vi "Lab Panel V5.22.vi"() -> ()   [LabVIEW 2013] (continued)
                    n1469 = Greater Or Equal?(x=w2760, y=w2759) -> (x >= y?=w2761:bool)
                    n1470 = case shown="True" w2761 {
                      tunnel: w2757 -> [w2764 _]
                      tunnel: w2756 -> [w2763 _]
                      tunnel: w2755 -> [w2762 _]
                      frame True {
                        n1471 = stacked-sequence {
                          tunnel: w2764 -> [w2767 _]
                          tunnel: w2763 -> [_ w2772]
                          tunnel: w2762 -> [w2765 _]
                          frame #0 {
                            n1472 = Build Array("T-RISE") -> (w2769:string[])
                            n1473 = Build Array(w2767) -> (w2768:dbl[])
                            n1474 = TDMS Write(0:w2765, 5:"TEST PASS", 7:w2769, 9:w2768) -> (15:w2771:errorcluster)  [unwired: 2 in, 3 out]
                            n1475 = local write "data file error"(w2771) -> ()
                          }
                          frame #1 {
                            n1476 = Bundle(cluster=w2772, "STATUS"="T-RISE PASS") -> (w2774:T4)  [unwired: 2 in]
                            n1477 = local write "RESULT LAB05-1"(TRUE) -> ()
                            n1478 = local write "DISP LAB05-1"(w2774) -> ()
                          }
                        }
                      }
                      frame False {
                      }
                    }
                  }
                }
              }
              frame #9 {
                # "LAB05-2"
                n1479 = Equal?(x=w2777, y=2) -> (x = y?=w2780:bool)
                n1480 = local read "DISP LAB05-2"() -> (w2782:T4)
                n1481 = Unbundle(w2782) -> ("STATUS"=w2783:string)  [unwired: 2 out]
                n1482 = Equal?(x=w2783, y="RUN") -> (x = y?=w2779:bool)
                n1483 = And(x=w2779, y=w2780) -> (x .and. y?=w2778:bool)
                n1484 = case shown="True" w2778 {
                  tunnel: w2782 -> [_ w2786]
                  tunnel: w2776 -> [_ w2789]
                  frame False {
                  }
                  frame True {
                    n1485 = local read "SET LAB05-2"() -> (w2788:T5)
                    n1486 = local read "TDMS LAB05-2"() -> (w2785:refnum<k34>)
                    n1487 = Unbundle(w2786) -> ("CYCLE"=w2790:dbl)  [unwired: 2 out]
                    n1488 = Unbundle(w2788) -> ("T-RISE mins"=w2787:dbl)  [unwired: 4 out]
                    n1489 = Greater Or Equal?(x=w2790, y=w2789) -> (x >= y?=w2791:bool)
                    n1490 = case shown="True" w2791 {
                      tunnel: w2787 -> [w2794 _]
                      tunnel: w2786 -> [w2793 _]
                      tunnel: w2785 -> [w2792 _]
                      frame True {
                        n1491 = stacked-sequence {
                          tunnel: w2794 -> [w2797 _]
                          tunnel: w2793 -> [_ w2802]
                          tunnel: w2792 -> [w2795 _]
                          frame #0 {
                            n1492 = Build Array("T-RISE") -> (w2799:string[])
                            n1493 = Build Array(w2797) -> (w2798:dbl[])
                            n1494 = TDMS Write(0:w2795, 5:"TEST PASS", 7:w2799, 9:w2798) -> (15:w2801:errorcluster)  [unwired: 2 in, 3 out]
                            n1495 = local write "data file error"(w2801) -> ()
                          }
                          frame #1 {
                            n1496 = Bundle(cluster=w2802, "STATUS"="T-RISE PASS") -> (w2804:T4)  [unwired: 2 in]
                            n1497 = local write "RESULT LAB05-2"(TRUE) -> ()
                            n1498 = local write "DISP LAB05-2"(w2804) -> ()
                          }
                        }
                      }
                      frame False {
                      }
                    }
                  }
                }
              }
            }
          }
          frame #6 {
            # "end test & close test files"
            n1499 = local read "MAIL SETTINGS"() -> (w2810:T7)
            n1500 = Unbundle(w2810) -> ("OUT SERVER ADDRESS"=w2809:string, "FROM ACCOUNT"=w2808:string)  [unwired: 5 out]
            n1501 = stacked-sequence {
              tunnel: w2820 -> [_ _ _ _ _ _ _ _ _ _]
              tunnel: w2821 -> [_ _ _ _ _ _ _ _ _ _]
              tunnel: w2819 -> [_ _ _ _ _ _ _ _ _ _]
              tunnel: w2818 -> [_ _ _ _ _ _ _ _ _ _]
              tunnel: w2817 -> [_ _ _ _ _ _ _ _ _ _]
              tunnel: w2816 -> [_ _ _ _ _ _ _ _ _ _]
              tunnel: w2815 -> [_ _ _ _ _ _ _ _ _ _]
              tunnel: w2814 -> [_ _ _ _ _ _ _ _ _ _]
              tunnel: w2813 -> [_ _ _ _ _ _ _ _ _ _]
              tunnel: w2812 -> [_ _ _ _ _ _ _ _ _ _]
              tunnel: w2809 -> [w2825 w2877 w2925 w2972 w3019 w3066 w3113 w3160 w3207 w3254]
              tunnel: w2808 -> [w2824 w2876 w2924 w2971 w3018 w3065 w3112 w3159 w3206 w3253]
              tunnel: "Mail Test File To:" -> [w2823 w2875 w2923 w2970 w3017 w3064 w3111 w3158 w3205 w3252]
              tunnel: "Mail Test Fail" -> [w2822 w2874 w2922 w2969 w3016 w3063 w3110 w3157 w3204 w3251]
              frame #0 {
                # "LAB01-1"
                n1502 = local read "DISP LAB01-1"() -> (w2829:T4)
                n1503 = local read "run lab01-1"() -> (w2826:bool)
                n1504 = local read "TDMS LAB01-1"() -> (w2827:refnum<k34>)
                n1505 = Unbundle(w2829) -> ("CYCLE"=w2830:dbl, "STATUS"=w2828:string)  [unwired: 1 out]
                n1506 = case shown="True" w2826 {
                  tunnel: w2830 -> [_ w2836]
                  tunnel: w2829 -> [_ w2838]
                  tunnel: w2828 -> [_ w2835]
                  tunnel: w2827 -> [_ w2837]
                  tunnel: w2825 -> [_ w2834]
                  tunnel: w2824 -> [_ w2833]
                  tunnel: w2823 -> [_ w2832]
                  tunnel: w2822 -> [_ w2831]
                  frame False {
                  }
                  frame True {
                    n1507 = Not Equal?(x=w2835, y="RUN") -> (x != y?=w2839:bool)
                    n1508 = Greater?(x=w2836, y=2.0) -> (0:w2841:bool)
                    n1509 = And(x=w2841, y=w2839) -> (x .and. y?=w2840:bool)
                    n1510 = case shown="True" w2840 {
                      tunnel: w2838 -> [_ w2851]
                      tunnel: w2837 -> [_ w2850]
                      tunnel: w2836 -> [_ w2849]
                      tunnel: w2835 -> [_ w2848]
                      tunnel: w2834 -> [_ w2847]
                      tunnel: w2833 -> [_ w2846]
                      tunnel: w2832 -> [_ w2845]
                      tunnel: w2831 -> [_ w2844]
                      frame False {
                      }
                      frame True {
                        n1511 = stacked-sequence {
                          tunnel: w2851 -> [w2855 _ _]
                          tunnel: w2850 -> [_ w2857 _]
                          tunnel: w2849 -> [_ _ _]
                          tunnel: w2848 -> [_ _ w2863]
                          tunnel: w2847 -> [_ _ w2862]
                          tunnel: w2846 -> [_ _ w2861]
                          tunnel: w2845 -> [_ _ w2860]
                          tunnel: w2844 -> [_ _ w2859]
                          frame #0 {
                            w2852 = FALSE
                            n1512 = local write "mail control"("END") -> ()
                            n1513 = Bundle(cluster=w2855) -> (w2854:T4)  [unwired: 3 in]
                            n1514 = local write "DISP LAB01-1"(w2854) -> ()
                            n1515 = local write "O/I  LAB01-1"(w2852) -> ()
                            n1516 = local write "run lab01-1"(w2852) -> ()
                            n1517 = local write "RUN LAB01-1"(w2852) -> ()
                          }
                          frame #1 {
                            n1518 = TDMS Close(11:w2857) -> (0:w2856:errorcluster)  [unwired: 1 in, 1 out]
                            n1519 = local write "data file error"(w2856) -> ()
                          }
                          frame #2 {
                            n1520 = stacked-sequence {
                              tunnel: "LAB01-1" -> [w2865 w2867 _]
                              tunnel: w2863 -> [_ w2873 _]
                              tunnel: w2862 -> [_ w2872 _]
                              tunnel: w2861 -> [_ w2871 _]
                              tunnel: w2860 -> [_ w2870 _]
                              tunnel: w2859 -> [_ w2869 _]
                              frame #0 {
                                n1521 = call "sub vi - defrag tdms v1.vi"("panel id"=w2865) -> ("error out"=w2864:errorcluster)  [unwired: 10 in]
                                n1522 = local write "data file error"(w2864) -> ()
                              }
                              frame #1 {
                                n1523 = Bundle("STATUS"=w2873, "OUT SERVER ADDRESS"=w2872, "FROM ACCOUNT"=w2871, "Mail Test File To:"=w2870, "Mail Test Fail"=w2869) -> (w2866:T25)  [unwired: 1 in]
                                n1524 = call "Save data file (pass-fail) v5.vi"("Input Cluster"=w2866, "panel id"=w2867) -> ("network file save error"=w2868:errorcluster)  [unwired: 8 in, 1 out]
                                n1525 = local write "data file error"(w2868) -> ()
                              }
                              frame #2 {
                              }
                            }
                          }
                        }
                      }
                    }
                  }
                }
              }
              frame #1 {
                # "LAB01-2"
                n1526 = local read "run lab01-2"() -> (w2878:bool)
                n1527 = case shown="True" w2878 {
                  tunnel: w2877 -> [_ w2882]
                  tunnel: w2876 -> [_ w2881]
                  tunnel: w2875 -> [_ w2880]
                  tunnel: w2874 -> [_ w2879]
                  frame False {
                  }
                  frame True {
                    n1528 = local read "DISP LAB01-2"() -> (w2890:T4)
                    n1529 = local read "TDMS LAB01-2"() -> (w2889:refnum<k34>)
                    n1530 = Unbundle(w2890) -> ("CYCLE"=w2884:dbl, "STATUS"=w2883:string)  [unwired: 1 out]
                    n1531 = Not Equal?(x=w2883, y="RUN") -> (x != y?=w2886:bool)
                    n1532 = Greater?(x=w2884, y=2.0) -> (0:w2887:bool)
                    n1533 = And(x=w2887, y=w2886) -> (x .and. y?=w2885:bool)
                    n1534 = case shown="True" w2885 {
                      tunnel: w2890 -> [_ w2899]
                      tunnel: w2889 -> [_ w2898]
                      tunnel: w2884 -> [_ w2897]
                      tunnel: w2883 -> [_ w2896]
                      tunnel: w2882 -> [_ w2895]
                      tunnel: w2881 -> [_ w2894]
                      tunnel: w2880 -> [_ w2893]
                      tunnel: w2879 -> [_ w2892]
                      frame False {
                      }
                      frame True {
                        n1535 = stacked-sequence {
                          tunnel: w2899 -> [w2902 _ _]
                          tunnel: w2898 -> [_ w2904 _]
                          tunnel: w2897 -> [_ _ _]
                          tunnel: w2896 -> [_ _ w2910]
                          tunnel: w2895 -> [_ _ w2909]
                          tunnel: w2894 -> [_ _ w2908]
                          tunnel: w2893 -> [_ _ w2907]
                          tunnel: w2892 -> [_ _ w2906]
                          frame #0 {
                            w2900 = FALSE
                            n1536 = local write "mail control"("END") -> ()
                            n1537 = Bundle(cluster=w2902) -> (w2903:T4)  [unwired: 3 in]
                            n1538 = local write "RUN LAB01-2"(w2900) -> ()
                            n1539 = local write "run lab01-2"(w2900) -> ()
                            n1540 = local write "O/I  LAB01-2"(w2900) -> ()
                            n1541 = local write "DISP LAB01-2"(w2903) -> ()
                          }
                          frame #1 {
                            n1542 = TDMS Close(11:w2904) -> (0:w2905:errorcluster)  [unwired: 1 in, 1 out]
                            n1543 = local write "data file error"(w2905) -> ()
                          }
                          frame #2 {
                            n1544 = stacked-sequence {
                              tunnel: "LAB01-2" -> [w2913 w2914]
                              tunnel: w2910 -> [_ w2919]
                              tunnel: w2909 -> [_ w2918]
                              tunnel: w2908 -> [_ w2917]
                              tunnel: w2907 -> [_ w2916]
                              tunnel: w2906 -> [_ w2915]
                              frame #0 {
                                n1545 = call "sub vi - defrag tdms v1.vi"("panel id"=w2913) -> ("error out"=w2912:errorcluster)  [unwired: 10 in]
                                n1546 = local write "data file error"(w2912) -> ()
                              }
                              frame #1 {
                                n1547 = Bundle("STATUS"=w2919, "OUT SERVER ADDRESS"=w2918, "FROM ACCOUNT"=w2917, "Mail Test File To:"=w2916, "Mail Test Fail"=w2915) -> (w2921:T25)  [unwired: 1 in]
                                n1548 = call "Save data file (pass-fail) v5.vi"("Input Cluster"=w2921, "panel id"=w2914) -> ("network file save error"=w2920:errorcluster)  [unwired: 8 in, 1 out]
                                n1549 = local write "data file error"(w2920) -> ()
                              }
                            }
                          }
                        }
                      }
                    }
                  }
                }
              }
              frame #2 {
                # "LAB02-1"
                n1550 = local read "run lab02-1"() -> (w2926:bool)
                n1551 = case shown="True" w2926 {
                  tunnel: w2925 -> [_ w2930]
                  tunnel: w2924 -> [_ w2929]
                  tunnel: w2923 -> [_ w2928]
                  tunnel: w2922 -> [_ w2927]
                  frame False {
                  }
                  frame True {
                    n1552 = local read "DISP LAB02-1"() -> (w2938:T4)
                    n1553 = Unbundle(w2938) -> ("CYCLE"=w2934:dbl, "STATUS"=w2931:string)  [unwired: 1 out]
                    n1554 = local read "TDMS LAB02-1"() -> (w2937:refnum<k34>)
                    n1555 = Not Equal?(x=w2931, y="RUN") -> (x != y?=w2933:bool)
                    n1556 = Greater?(x=w2934, y=2.0) -> (0:w2935:bool)
                    n1557 = And(x=w2935, y=w2933) -> (x .and. y?=w2932:bool)
                    n1558 = case shown="True" w2932 {
                      tunnel: w2938 -> [_ w2946]
                      tunnel: w2937 -> [_ w2945]
                      tunnel: w2931 -> [_ w2944]
                      tunnel: w2930 -> [_ w2943]
                      tunnel: w2929 -> [_ w2942]
                      tunnel: w2928 -> [_ w2941]
                      tunnel: w2927 -> [_ w2940]
                      frame False {
                      }
                      frame True {
                        n1559 = stacked-sequence {
                          tunnel: w2946 -> [w2949 _ _]
                          tunnel: w2945 -> [_ w2951 _]
                          tunnel: w2944 -> [_ _ w2957]
                          tunnel: w2943 -> [_ _ w2956]
                          tunnel: w2942 -> [_ _ w2955]
                          tunnel: w2941 -> [_ _ w2954]
                          tunnel: w2940 -> [_ _ w2953]
                          frame #0 {
                            w2947 = FALSE
                            n1560 = local write "mail control"("END") -> ()
                            n1561 = Bundle(cluster=w2949) -> (w2950:T4)  [unwired: 3 in]
                            n1562 = local write "O/I  LAB02-1"(w2947) -> ()
                            n1563 = local write "RUN LAB02-1"(w2947) -> ()
                            n1564 = local write "run lab02-1"(w2947) -> ()
                            n1565 = local write "DISP LAB02-1"(w2950) -> ()
                          }
                          frame #1 {
                            n1566 = TDMS Close(11:w2951) -> (0:w2952:errorcluster)  [unwired: 1 in, 1 out]
                            n1567 = local write "data file error"(w2952) -> ()
                          }
                          frame #2 {
                            n1568 = stacked-sequence {
                              tunnel: "LAB02-1" -> [w2960 w2967]
                              tunnel: w2957 -> [_ w2965]
                              tunnel: w2956 -> [_ w2964]
                              tunnel: w2955 -> [_ w2963]
                              tunnel: w2954 -> [_ w2962]
                              tunnel: w2953 -> [_ w2961]
                              frame #0 {
                                n1569 = call "sub vi - defrag tdms v1.vi"("panel id"=w2960) -> ("error out"=w2959:errorcluster)  [unwired: 10 in]
                                n1570 = local write "data file error"(w2959) -> ()
                              }
                              frame #1 {
                                n1571 = Bundle("STATUS"=w2965, "OUT SERVER ADDRESS"=w2964, "FROM ACCOUNT"=w2963, "Mail Test File To:"=w2962, "Mail Test Fail"=w2961) -> (w2966:T25)  [unwired: 1 in]
                                n1572 = call "Save data file (pass-fail) v5.vi"("Input Cluster"=w2966, "panel id"=w2967) -> ("network file save error"=w2968:errorcluster)  [unwired: 8 in, 1 out]
                                n1573 = local write "data file error"(w2968) -> ()
                              }
                            }
                          }
                        }
                      }
                    }
                  }
                }
              }
              frame #3 {
                # "LAB02-2"
                n1574 = local read "run lab02-2"() -> (w2973:bool)
                n1575 = case shown="True" w2973 {
                  tunnel: w2972 -> [_ w2977]
                  tunnel: w2971 -> [_ w2976]
                  tunnel: w2970 -> [_ w2975]
                  tunnel: w2969 -> [_ w2974]
                  frame False {
                  }
                  frame True {
                    n1576 = local read "DISP LAB02-2"() -> (w2985:T4)
                    n1577 = local read "TDMS LAB02-2"() -> (w2984:refnum<k34>)
                    n1578 = Unbundle(w2985) -> ("CYCLE"=w2981:dbl, "STATUS"=w2978:string)  [unwired: 1 out]
                    n1579 = Not Equal?(x=w2978, y="RUN") -> (x != y?=w2980:bool)
                    n1580 = Greater?(x=w2981, y=2.0) -> (0:w2982:bool)
                    n1581 = And(x=w2982, y=w2980) -> (x .and. y?=w2979:bool)
                    n1582 = case shown="True" w2979 {
                      tunnel: w2985 -> [_ w2993]
                      tunnel: w2984 -> [_ w2992]
                      tunnel: w2978 -> [_ w2991]
                      tunnel: w2977 -> [_ w2990]
                      tunnel: w2976 -> [_ w2989]
                      tunnel: w2975 -> [_ w2988]
                      tunnel: w2974 -> [_ w2987]
                      frame False {
                      }
                      frame True {
                        n1583 = stacked-sequence {
                          tunnel: w2993 -> [w2996 _ _]
                          tunnel: w2992 -> [_ w2998 _]
                          tunnel: w2991 -> [_ _ w3004]
                          tunnel: w2990 -> [_ _ w3003]
                          tunnel: w2989 -> [_ _ w3002]
                          tunnel: w2988 -> [_ _ w3001]
                          tunnel: w2987 -> [_ _ w3000]
                          frame #0 {
                            w2994 = FALSE
                            n1584 = local write "mail control"("END") -> ()
                            n1585 = Bundle(cluster=w2996) -> (w2997:T4)  [unwired: 3 in]
                            n1586 = local write "O/I  LAB02-2"(w2994) -> ()
                            n1587 = local write "run lab02-2"(w2994) -> ()
                            n1588 = local write "RUN LAB02-2"(w2994) -> ()
                            n1589 = local write "DISP LAB02-2"(w2997) -> ()
                          }
                          frame #1 {
                            n1590 = TDMS Close(11:w2998) -> (0:w2999:errorcluster)  [unwired: 1 in, 1 out]
                            n1591 = local write "data file error"(w2999) -> ()
                          }
                          frame #2 {
                            n1592 = stacked-sequence {
                              tunnel: "LAB02-2" -> [w3007 w3013]
                              tunnel: w3004 -> [_ w3012]
                              tunnel: w3003 -> [_ w3011]
                              tunnel: w3002 -> [_ w3010]
                              tunnel: w3001 -> [_ w3009]
                              tunnel: w3000 -> [_ w3008]
                              frame #0 {
                                n1593 = call "sub vi - defrag tdms v1.vi"("panel id"=w3007) -> ("error out"=w3006:errorcluster)  [unwired: 10 in]
                                n1594 = local write "data file error"(w3006) -> ()
                              }
                              frame #1 {
                                n1595 = Bundle("STATUS"=w3012, "OUT SERVER ADDRESS"=w3011, "FROM ACCOUNT"=w3010, "Mail Test File To:"=w3009, "Mail Test Fail"=w3008) -> (w3015:T25)  [unwired: 1 in]
                                n1596 = call "Save data file (pass-fail) v5.vi"("Input Cluster"=w3015, "panel id"=w3013) -> ("network file save error"=w3014:errorcluster)  [unwired: 8 in, 1 out]
                                n1597 = local write "data file error"(w3014) -> ()
                              }
                            }
                          }
                        }
                      }
                    }
                  }
                }
              }
              frame #4 {
                # "LAB03-1"
                n1598 = local read "run lab03-1"() -> (w3020:bool)
                n1599 = case shown="True" w3020 {
                  tunnel: w3019 -> [_ w3024]
                  tunnel: w3018 -> [_ w3023]
                  tunnel: w3017 -> [_ w3022]
                  tunnel: w3016 -> [_ w3021]
                  frame False {
                  }
                  frame True {
                    n1600 = local read "DISP LAB03-1"() -> (w3032:T4)
                    n1601 = local read "TDMS LAB03-1"() -> (w3031:refnum<k34>)
                    n1602 = Unbundle(w3032) -> ("CYCLE"=w3028:dbl, "STATUS"=w3025:string)  [unwired: 1 out]
                    n1603 = Not Equal?(x=w3025, y="RUN") -> (x != y?=w3027:bool)
                    n1604 = Greater?(x=w3028, y=2.0) -> (0:w3029:bool)
                    n1605 = And(x=w3029, y=w3027) -> (x .and. y?=w3026:bool)
                    n1606 = case shown="True" w3026 {
                      tunnel: w3032 -> [_ w3040]
                      tunnel: w3031 -> [_ w3039]
                      tunnel: w3025 -> [_ w3038]
                      tunnel: w3024 -> [_ w3037]
                      tunnel: w3023 -> [_ w3036]
                      tunnel: w3022 -> [_ w3035]
                      tunnel: w3021 -> [_ w3034]
                      frame False {
                      }
                      frame True {
                        n1607 = stacked-sequence {
                          tunnel: w3040 -> [w3043 _ _]
                          tunnel: w3039 -> [_ w3045 _]
                          tunnel: w3038 -> [_ _ w3051]
                          tunnel: w3037 -> [_ _ w3050]
                          tunnel: w3036 -> [_ _ w3049]
                          tunnel: w3035 -> [_ _ w3048]
                          tunnel: w3034 -> [_ _ w3047]
                          frame #0 {
                            w3041 = FALSE
                            n1608 = local write "mail control"("END") -> ()
                            n1609 = Bundle(cluster=w3043) -> (w3044:T4)  [unwired: 3 in]
                            n1610 = local write "O/I  LAB03-1"(w3041) -> ()
                            n1611 = local write "run lab03-1"(w3041) -> ()
                            n1612 = local write "RUN LAB03-1"(w3041) -> ()
                            n1613 = local write "DISP LAB03-1"(w3044) -> ()
                          }
                          frame #1 {
                            n1614 = TDMS Close(11:w3045) -> (0:w3046:errorcluster)  [unwired: 1 in, 1 out]
                            n1615 = local write "data file error"(w3046) -> ()
                          }
                          frame #2 {
                            n1616 = stacked-sequence {
                              tunnel: "LAB03-1" -> [w3054 w3060]
                              tunnel: w3051 -> [_ w3059]
                              tunnel: w3050 -> [_ w3058]
                              tunnel: w3049 -> [_ w3057]
                              tunnel: w3048 -> [_ w3056]
                              tunnel: w3047 -> [_ w3055]
                              frame #0 {
                                n1617 = call "sub vi - defrag tdms v1.vi"("panel id"=w3054) -> ("error out"=w3053:errorcluster)  [unwired: 10 in]
                                n1618 = local write "data file error"(w3053) -> ()
                              }
                              frame #1 {
                                n1619 = Bundle("STATUS"=w3059, "OUT SERVER ADDRESS"=w3058, "FROM ACCOUNT"=w3057, "Mail Test File To:"=w3056, "Mail Test Fail"=w3055) -> (w3062:T25)  [unwired: 1 in]
                                n1620 = call "Save data file (pass-fail) v5.vi"("Input Cluster"=w3062, "panel id"=w3060) -> ("network file save error"=w3061:errorcluster)  [unwired: 8 in, 1 out]
                                n1621 = local write "data file error"(w3061) -> ()
                              }
                            }
                          }
                        }
                      }
                    }
                  }
                }
              }
              frame #5 {
                # "LAB03-2"
                n1622 = local read "run lab03-2"() -> (w3067:bool)
                n1623 = case shown="True" w3067 {
                  tunnel: w3066 -> [_ w3071]
                  tunnel: w3065 -> [_ w3070]
                  tunnel: w3064 -> [_ w3069]
                  tunnel: w3063 -> [_ w3068]
                  frame False {
                  }
                  frame True {
                    n1624 = local read "DISP LAB03-2"() -> (w3079:T4)
                    n1625 = Unbundle(w3079) -> ("CYCLE"=w3075:dbl, "STATUS"=w3072:string)  [unwired: 1 out]
                    n1626 = local read "TDMS LAB03-2"() -> (w3078:refnum<k34>)
                    n1627 = Not Equal?(x=w3072, y="RUN") -> (x != y?=w3074:bool)
                    n1628 = Greater?(x=w3075, y=2.0) -> (0:w3076:bool)
                    n1629 = And(x=w3076, y=w3074) -> (x .and. y?=w3073:bool)
                    n1630 = case shown="True" w3073 {
                      tunnel: w3079 -> [_ w3087]
                      tunnel: w3078 -> [_ w3086]
                      tunnel: w3072 -> [_ w3085]
                      tunnel: w3071 -> [_ w3084]
                      tunnel: w3070 -> [_ w3083]
                      tunnel: w3069 -> [_ w3082]
                      tunnel: w3068 -> [_ w3081]
                      frame False {
                      }
                      frame True {
                        n1631 = stacked-sequence {
                          tunnel: w3087 -> [w3090 _ _]
                          tunnel: w3086 -> [_ w3092 _]
                          tunnel: w3085 -> [_ _ w3098]
                          tunnel: w3084 -> [_ _ w3097]
                          tunnel: w3083 -> [_ _ w3096]
                          tunnel: w3082 -> [_ _ w3095]
                          tunnel: w3081 -> [_ _ w3094]
                          frame #0 {
                            w3088 = FALSE
                            n1632 = local write "mail control"("END") -> ()
                            n1633 = Bundle(cluster=w3090) -> (w3091:T4)  [unwired: 3 in]
                            n1634 = local write "RUN LAB03-2"(w3088) -> ()
                            n1635 = local write "O/I  LAB03-2"(w3088) -> ()
                            n1636 = local write "DISP LAB03-2"(w3091) -> ()
                            n1637 = local write "run lab03-2"(w3088) -> ()
                          }
                          frame #1 {
                            n1638 = TDMS Close(11:w3092) -> (0:w3093:errorcluster)  [unwired: 1 in, 1 out]
                            n1639 = local write "data file error"(w3093) -> ()
                          }
                          frame #2 {
                            n1640 = stacked-sequence {
                              tunnel: "LAB03-2" -> [w3101 w3102]
                              tunnel: w3098 -> [_ w3107]
                              tunnel: w3097 -> [_ w3106]
                              tunnel: w3096 -> [_ w3105]
                              tunnel: w3095 -> [_ w3104]
                              tunnel: w3094 -> [_ w3103]
                              frame #0 {
                                n1641 = call "sub vi - defrag tdms v1.vi"("panel id"=w3101) -> ("error out"=w3100:errorcluster)  [unwired: 10 in]
                                n1642 = local write "data file error"(w3100) -> ()
                              }
                              frame #1 {
                                n1643 = Bundle("STATUS"=w3107, "OUT SERVER ADDRESS"=w3106, "FROM ACCOUNT"=w3105, "Mail Test File To:"=w3104, "Mail Test Fail"=w3103) -> (w3109:T25)  [unwired: 1 in]
                                n1644 = call "Save data file (pass-fail) v5.vi"("Input Cluster"=w3109, "panel id"=w3102) -> ("network file save error"=w3108:errorcluster)  [unwired: 8 in, 1 out]
                                n1645 = local write "data file error"(w3108) -> ()
                              }
                            }
                          }
                        }
                      }
                    }
                  }
                }
              }
              frame #6 {
                # "LAB04-1"
                n1646 = local read "run lab04-1"() -> (w3114:bool)
                n1647 = case shown="True" w3114 {
                  tunnel: w3113 -> [_ w3118]
                  tunnel: w3112 -> [_ w3117]
                  tunnel: w3111 -> [_ w3116]
                  tunnel: w3110 -> [_ w3115]
                  frame False {
                  }
                  frame True {
                    n1648 = local read "DISP LAB04-1"() -> (w3126:T4)
                    n1649 = Unbundle(w3126) -> ("CYCLE"=w3122:dbl, "STATUS"=w3119:string)  [unwired: 1 out]
                    n1650 = local read "TDMS LAB04-1"() -> (w3125:refnum<k34>)
                    n1651 = Not Equal?(x=w3119, y="RUN") -> (x != y?=w3121:bool)
                    n1652 = Greater?(x=w3122, y=2.0) -> (0:w3123:bool)
                    n1653 = And(x=w3123, y=w3121) -> (x .and. y?=w3120:bool)
                    n1654 = case shown="True" w3120 {
                      tunnel: w3126 -> [_ w3134]
                      tunnel: w3125 -> [_ w3133]
                      tunnel: w3119 -> [_ w3132]
                      tunnel: w3118 -> [_ w3131]
                      tunnel: w3117 -> [_ w3130]
                      tunnel: w3116 -> [_ w3129]
                      tunnel: w3115 -> [_ w3128]
                      frame False {
                      }
                      frame True {
                        n1655 = stacked-sequence {
                          tunnel: w3134 -> [w3137 _ _]
                          tunnel: w3133 -> [_ w3139 _]
                          tunnel: w3132 -> [_ _ w3145]
                          tunnel: w3131 -> [_ _ w3144]
                          tunnel: w3130 -> [_ _ w3143]
                          tunnel: w3129 -> [_ _ w3142]
                          tunnel: w3128 -> [_ _ w3141]
                          frame #0 {
                            w3135 = FALSE
                            n1656 = local write "mail control"("END") -> ()
                            n1657 = Bundle(cluster=w3137) -> (w3138:T4)  [unwired: 3 in]
                            n1658 = local write "RUN LAB04-1"(w3135) -> ()
                            n1659 = local write "O/I  LAB04-1"(w3135) -> ()
                            n1660 = local write "run lab04-1"(w3135) -> ()
                            n1661 = local write "DISP LAB04-1"(w3138) -> ()
                          }
                          frame #1 {
                            n1662 = TDMS Close(11:w3139) -> (0:w3140:errorcluster)  [unwired: 1 in, 1 out]
                            n1663 = local write "data file error"(w3140) -> ()
                          }
                          frame #2 {
                            n1664 = stacked-sequence {
                              tunnel: "LAB04-1" -> [w3148 w3149]
                              tunnel: w3145 -> [_ w3154]
                              tunnel: w3144 -> [_ w3153]
                              tunnel: w3143 -> [_ w3152]
                              tunnel: w3142 -> [_ w3151]
                              tunnel: w3141 -> [_ w3150]
                              frame #0 {
                                n1665 = call "sub vi - defrag tdms v1.vi"("panel id"=w3148) -> ("error out"=w3147:errorcluster)  [unwired: 10 in]
                                n1666 = local write "data file error"(w3147) -> ()
                              }
                              frame #1 {
                                n1667 = Bundle("STATUS"=w3154, "OUT SERVER ADDRESS"=w3153, "FROM ACCOUNT"=w3152, "Mail Test File To:"=w3151, "Mail Test Fail"=w3150) -> (w3156:T25)  [unwired: 1 in]
                                n1668 = call "Save data file (pass-fail) v5.vi"("Input Cluster"=w3156, "panel id"=w3149) -> ("network file save error"=w3155:errorcluster)  [unwired: 8 in, 1 out]
                                n1669 = local write "data file error"(w3155) -> ()
                              }
                            }
                          }
                        }
                      }
                    }
                  }
                }
              }
              frame #7 {
                # "LAB04-2"
                n1670 = local read "run lab04-2"() -> (w3161:bool)
                n1671 = case shown="True" w3161 {
                  tunnel: w3160 -> [_ w3165]
                  tunnel: w3159 -> [_ w3164]
                  tunnel: w3158 -> [_ w3163]
                  tunnel: w3157 -> [_ w3162]
                  frame False {
                  }
                  frame True {
                    n1672 = local read "DISP LAB04-2"() -> (w3173:T4)
                    n1673 = Unbundle(w3173) -> ("CYCLE"=w3169:dbl, "STATUS"=w3166:string)  [unwired: 1 out]
                    n1674 = Not Equal?(x=w3166, y="RUN") -> (x != y?=w3168:bool)
                    n1675 = local read "TDMS LAB04-2"() -> (w3172:refnum<k34>)
                    n1676 = Greater?(x=w3169, y=2.0) -> (0:w3170:bool)
                    n1677 = And(x=w3170, y=w3168) -> (x .and. y?=w3167:bool)
                    n1678 = case shown="True" w3167 {
                      tunnel: w3173 -> [_ w3181]
                      tunnel: w3172 -> [_ w3180]
                      tunnel: w3166 -> [_ w3179]
                      tunnel: w3165 -> [_ w3178]
                      tunnel: w3164 -> [_ w3177]
                      tunnel: w3163 -> [_ w3176]
                      tunnel: w3162 -> [_ w3175]
                      frame False {
                      }
                      frame True {
                        n1679 = stacked-sequence {
                          tunnel: w3181 -> [w3184 _ _]
                          tunnel: w3180 -> [_ w3186 _]
                          tunnel: w3179 -> [_ _ w3192]
                          tunnel: w3178 -> [_ _ w3191]
                          tunnel: w3177 -> [_ _ w3190]
                          tunnel: w3176 -> [_ _ w3189]
                          tunnel: w3175 -> [_ _ w3188]
                          frame #0 {
                            w3182 = FALSE
                            n1680 = local write "mail control"("END") -> ()
                            n1681 = Bundle(cluster=w3184) -> (w3185:T4)  [unwired: 3 in]
                            n1682 = local write "O/I  LAB04-2"(w3182) -> ()
                            n1683 = local write "RUN LAB04-2"(w3182) -> ()
                            n1684 = local write "run lab04-2"(w3182) -> ()
                            n1685 = local write "DISP LAB04-2"(w3185) -> ()
                          }
                          frame #1 {
                            n1686 = TDMS Close(11:w3186) -> (0:w3187:errorcluster)  [unwired: 1 in, 1 out]
                            n1687 = local write "data file error"(w3187) -> ()
                          }
                          frame #2 {
                            n1688 = stacked-sequence {
                              tunnel: "LAB04-2" -> [w3195 w3196]
                              tunnel: w3192 -> [_ w3201]
                              tunnel: w3191 -> [_ w3200]
                              tunnel: w3190 -> [_ w3199]
                              tunnel: w3189 -> [_ w3198]
                              tunnel: w3188 -> [_ w3197]
                              frame #0 {
                                n1689 = call "sub vi - defrag tdms v1.vi"("panel id"=w3195) -> ("error out"=w3194:errorcluster)  [unwired: 10 in]
                                n1690 = local write "data file error"(w3194) -> ()
                              }
                              frame #1 {
                                n1691 = Bundle("STATUS"=w3201, "OUT SERVER ADDRESS"=w3200, "FROM ACCOUNT"=w3199, "Mail Test File To:"=w3198, "Mail Test Fail"=w3197) -> (w3203:T25)  [unwired: 1 in]
                                n1692 = call "Save data file (pass-fail) v5.vi"("Input Cluster"=w3203, "panel id"=w3196) -> ("network file save error"=w3202:errorcluster)  [unwired: 8 in, 1 out]
                                n1693 = local write "data file error"(w3202) -> ()
                              }
                            }
                          }
                        }
                      }
                    }
                  }
                }
              }
              frame #8 {
                # "LAB05-1"
                n1694 = local read "run lab05-1"() -> (w3208:bool)
                n1695 = case shown="True" w3208 {
                  tunnel: w3207 -> [_ w3212]
                  tunnel: w3206 -> [_ w3211]
                  tunnel: w3205 -> [_ w3210]
                  tunnel: w3204 -> [_ w3209]
                  frame False {
                  }
                  frame True {
                    n1696 = local read "DISP LAB05-1"() -> (w3220:T4)
                    n1697 = Unbundle(w3220) -> ("CYCLE"=w3216:dbl, "STATUS"=w3213:string)  [unwired: 1 out]
                    n1698 = Not Equal?(x=w3213, y="RUN") -> (x != y?=w3215:bool)
                    n1699 = local read "TDMS LAB05-1"() -> (w3219:refnum<k34>)
                    n1700 = Greater?(x=w3216, y=2.0) -> (0:w3217:bool)
                    n1701 = And(x=w3217, y=w3215) -> (x .and. y?=w3214:bool)
                    n1702 = case shown="True" w3214 {
                      tunnel: w3220 -> [_ w3228]
                      tunnel: w3219 -> [_ w3227]
                      tunnel: w3213 -> [_ w3226]
                      tunnel: w3212 -> [_ w3225]
                      tunnel: w3211 -> [_ w3224]
                      tunnel: w3210 -> [_ w3223]
                      tunnel: w3209 -> [_ w3222]
                      frame False {
                      }
                      frame True {
                        n1703 = stacked-sequence {
                          tunnel: w3228 -> [w3231 _ _]
                          tunnel: w3227 -> [_ w3233 _]
                          tunnel: w3226 -> [_ _ w3239]
                          tunnel: w3225 -> [_ _ w3238]
                          tunnel: w3224 -> [_ _ w3237]
                          tunnel: w3223 -> [_ _ w3236]
                          tunnel: w3222 -> [_ _ w3235]
                          frame #0 {
                            w3229 = FALSE
                            n1704 = local write "mail control"("END") -> ()
                            n1705 = Bundle(cluster=w3231) -> (w3232:T4)  [unwired: 3 in]
                            n1706 = local write "O/I  LAB05-1"(w3229) -> ()
                            n1707 = local write "RUN LAB05-1"(w3229) -> ()
                            n1708 = local write "run lab05-1"(w3229) -> ()
                            n1709 = local write "DISP LAB05-1"(w3232) -> ()
                          }
                          frame #1 {
                            n1710 = TDMS Close(11:w3233) -> (0:w3234:errorcluster)  [unwired: 1 in, 1 out]
                            n1711 = local write "data file error"(w3234) -> ()
                          }
                          frame #2 {
                            n1712 = stacked-sequence {
                              tunnel: "LAB05-1" -> [w3242 w3248]
                              tunnel: w3239 -> [_ w3247]
                              tunnel: w3238 -> [_ w3246]
                              tunnel: w3237 -> [_ w3245]
                              tunnel: w3236 -> [_ w3244]
                              tunnel: w3235 -> [_ w3243]
                              frame #0 {
                                n1713 = call "sub vi - defrag tdms v1.vi"("panel id"=w3242) -> ("error out"=w3241:errorcluster)  [unwired: 10 in]
                                n1714 = local write "data file error"(w3241) -> ()
                              }
                              frame #1 {
                                n1715 = Bundle("STATUS"=w3247, "OUT SERVER ADDRESS"=w3246, "FROM ACCOUNT"=w3245, "Mail Test File To:"=w3244, "Mail Test Fail"=w3243) -> (w3250:T25)  [unwired: 1 in]
                                n1716 = call "Save data file (pass-fail) v5.vi"("Input Cluster"=w3250, "panel id"=w3248) -> ("network file save error"=w3249:errorcluster)  [unwired: 8 in, 1 out]
                                n1717 = local write "data file error"(w3249) -> ()
                              }
                            }
                          }
                        }
                      }
                    }
                  }
                }
              }
              frame #9 {
                # "LAB05-2"
                n1718 = local read "run lab05-2"() -> (w3255:bool)
                n1719 = case shown="True" w3255 {
                  tunnel: w3254 -> [_ w3259]
                  tunnel: w3253 -> [_ w3258]
                  tunnel: w3252 -> [_ w3257]
                  tunnel: w3251 -> [_ w3256]
                  frame False {
                  }
                  frame True {
                    n1720 = local read "DISP LAB05-2"() -> (w3267:T4)
                    n1721 = Unbundle(w3267) -> ("CYCLE"=w3263:dbl, "STATUS"=w3260:string)  [unwired: 1 out]
                    n1722 = Not Equal?(x=w3260, y="RUN") -> (x != y?=w3262:bool)
                    n1723 = local read "TDMS LAB05-2"() -> (w3266:refnum<k34>)
                    n1724 = Greater?(x=w3263, y=2.0) -> (0:w3264:bool)
                    n1725 = And(x=w3264, y=w3262) -> (x .and. y?=w3261:bool)
                    n1726 = case shown="True" w3261 {
                      tunnel: w3267 -> [_ w3275]
                      tunnel: w3266 -> [_ w3274]
                      tunnel: w3260 -> [_ w3273]
                      tunnel: w3259 -> [_ w3272]
                      tunnel: w3258 -> [_ w3271]
                      tunnel: w3257 -> [_ w3270]
                      tunnel: w3256 -> [_ w3269]
                      frame False {
                      }
                      frame True {
                        n1727 = stacked-sequence {
                          tunnel: w3275 -> [w3278 _ _]
                          tunnel: w3274 -> [_ w3280 _]
                          tunnel: w3273 -> [_ _ w3286]
                          tunnel: w3272 -> [_ _ w3285]
                          tunnel: w3271 -> [_ _ w3284]
                          tunnel: w3270 -> [_ _ w3283]
                          tunnel: w3269 -> [_ _ w3282]
                          frame #0 {
                            w3276 = FALSE
                            n1728 = local write "mail control"("END") -> ()
                            n1729 = Bundle(cluster=w3278) -> (w3279:T4)  [unwired: 3 in]
                            n1730 = local write "RUN LAB05-2"(w3276) -> ()
                            n1731 = local write "O/I  LAB05-2"(w3276) -> ()
                            n1732 = local write "run lab05-2"(w3276) -> ()
                            n1733 = local write "DISP LAB05-2"(w3279) -> ()
                          }
                          frame #1 {
                            n1734 = TDMS Close(11:w3280) -> (0:w3281:errorcluster)  [unwired: 1 in, 1 out]
                            n1735 = local write "data file error"(w3281) -> ()
                          }
                          frame #2 {
                            n1736 = stacked-sequence {
                              tunnel: "LAB05-2" -> [w3289 w3295]
                              tunnel: w3286 -> [_ w3294]
                              tunnel: w3285 -> [_ w3293]
                              tunnel: w3284 -> [_ w3292]
                              tunnel: w3283 -> [_ w3291]
                              tunnel: w3282 -> [_ w3290]
                              frame #0 {
                                n1737 = call "sub vi - defrag tdms v1.vi"("panel id"=w3289) -> ("error out"=w3288:errorcluster)  [unwired: 10 in]
                                n1738 = local write "data file error"(w3288) -> ()
                              }
                              frame #1 {
                                n1739 = Bundle("STATUS"=w3294, "OUT SERVER ADDRESS"=w3293, "FROM ACCOUNT"=w3292, "Mail Test File To:"=w3291, "Mail Test Fail"=w3290) -> (w3297:T25)  [unwired: 1 in]
                                n1740 = call "Save data file (pass-fail) v5.vi"("Input Cluster"=w3297, "panel id"=w3295) -> ("network file save error"=w3296:errorcluster)  [unwired: 8 in, 1 out]
                                n1741 = local write "data file error"(w3296) -> ()
                              }
                            }
                          }
                        }
                      }
                    }
                  }
                }
              }
            }
            n1742 = local read "Network Directory"() -> (w2811:path)
            n1743 = global write "Global 1.vi" "Network Drive"(w2811) -> ()
          }
          frame #7 {
            # "disable functions"
            n1744 = stacked-sequence {
              tunnel: w3307 -> [w3321 _ w3378]
              tunnel: w3306 -> [w3316 _ w3377]
              tunnel: w3305 -> [w3315 _ w3376]
              tunnel: w3304 -> [w3313 _ w3375]
              tunnel: w3303 -> [w3314 _ w3374]
              tunnel: w3302 -> [_ w3338 w3373]
              tunnel: w3301 -> [_ w3339 w3372]
              tunnel: w3300 -> [_ w3340 w3371]
              tunnel: w3299 -> [_ w3341 w3370]
              tunnel: w3298 -> [_ w3342 w3369]
              frame #0 {
                n1745 = Select(t=2, s=w3313, f=0) -> (s? t:f=w3309:i32)
                n1746 = Select(t=2, s=w3315, f=0) -> (s? t:f=w3310:i32)
                n1747 = Select(t=2, s=w3314, f=0) -> (s? t:f=w3308:i32)
                n1748 = Select(t=2, s=w3321, f=0) -> (s? t:f=w3312:i32)
                n1749 = Select(t=2, s=w3316, f=0) -> (s? t:f=w3311:i32)
                n1750 = property on="SELECT LAB02-2" class="RadioBtnsControl (strict)"("DisabledEnum"=w3309) -> ()  [unwired: 2 in, 2 out]
                n1751 = property on="SELECT LAB02-1" class="RadioBtnsControl (strict)"("DisabledEnum"=w3310) -> ()  [unwired: 2 in, 2 out]
                n1752 = property on="SELECT LAB03-1" class="RadioBtnsControl (strict)"("DisabledEnum"=w3308) -> ()  [unwired: 2 in, 2 out]
                n1753 = property on="SELECT LAB01-1" class="RadioBtnsControl (strict)"("DisabledEnum"=w3312) -> ()  [unwired: 2 in, 2 out]
                n1754 = property on="SELECT LAB01-2" class="RadioBtnsControl (strict)"("DisabledEnum"=w3311) -> ()  [unwired: 2 in, 2 out]
                n1755 = Not(x=w3321) -> (.not. x?=w3322:bool)
                n1756 = property on="RESULT LAB01-1" class="Bool (strict)"("Visible"=w3322) -> ()  [unwired: 2 in, 2 out]
                n1757 = Not(x=w3316) -> (.not. x?=w3320:bool)
                n1758 = Not(x=w3315) -> (.not. x?=w3319:bool)
                n1759 = Not(x=w3313) -> (.not. x?=w3318:bool)
                n1760 = property on="RESULT LAB01-2" class="Bool (strict)"("Visible"=w3320) -> ()  [unwired: 2 in, 2 out]
                n1761 = Not(x=w3314) -> (.not. x?=w3317:bool)
                n1762 = property on="RESULT LAB02-1" class="Bool (strict)"("Visible"=w3319) -> ()  [unwired: 2 in, 2 out]
                n1763 = property on="RESULT LAB02-2" class="Bool (strict)"("Visible"=w3318) -> ()  [unwired: 2 in, 2 out]
                n1764 = property on="RESULT LAB03-1" class="Bool (strict)"("Visible"=w3317) -> ()  [unwired: 2 in, 2 out]
                n1765 = property on="SET LAB01-1" class="Clust (strict)"("DisabledEnum"=w3312) -> ()  [unwired: 2 in, 2 out]
